vi "Initialize.vi"(8 "error in (no error)":errorcluster, 10 "CommandText":string, 11 "PathCommands.MoveTo in":refnum<class "PathCommands.MoveTo.lvclass">) -> (0 "error out":errorcluster, 3 "PathCommands.MoveTo out":refnum<class "PathCommands.MoveTo.lvclass">)   [LabVIEW 2019, in "PathCommands.MoveTo.lvclass"]
uses:
  PathCommands.MoveTo.lvclass
  PathCommands/PathCommands.lvclass
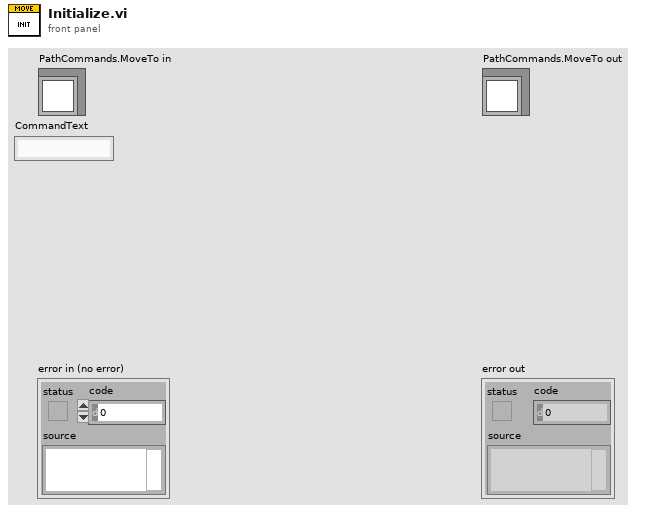
[diagram p1: front panel]
types:
  T1 = enum16{"None", "After", "Before", "Last", "First"}[]
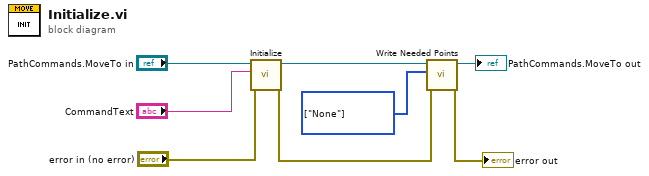
[diagram p0: block diagram]
diagram:
  w1 = T1 [enum."None"] items=["None", "After", "Before", "Last", "First"] ("Needed Points")
  n1 = call-parent "Initialize.vi"("error in (no error)"="error in (no error)", "CommandText"="CommandText", "PathCommands in"="PathCommands.MoveTo in") -> ("error out"=w3:errorcluster, "PathCommands out"=w5:refnum<class "PathCommands.MoveTo.lvclass">)  [unwired: 7 in]
  n2 = call-dynamic "Write Needed Points.vi"("error in (no error)"=w3, "Needed Points"=w1, "PathCommands in"=w5) -> ("error out"=→"error out":errorcluster, "PathCommands out"=→"PathCommands.MoveTo out":refnum<class "PathCommands.MoveTo.lvclass">)  [unwired: 7 in]
